vi "LDA_IP_NI-DAQmx.vi"(0 "Board type":T1=enum."NI-DAQmx", 1 "interval scanning":bool, 7 "Trigger mode":T2, 9 "output polarity":u16(ring)=1 items=["do not change", "positive", "negative"]) -> (3 "LDA Binary output":u16[][](array[numeric]), 6 "I16 TOF block (mu.s)":i16[](array[numeric])=[-338, -324, -346, -351, -326, -357, -344, -311, -375, -296], 15 "error out":errorcluster)   [LabVIEW 2012]
uses:
  Controls/Trigger_Mode.ctl
  Controls/Board_Types.ctl
  Controls/Block_start_and_end.ctl
  <vilib>/DAQmx/read.llb/DAQmx Read (Analog 2D DBL NChan NSamp).vi
  Globals/Meas_global.vi
  Globals/LDA_meas_global_1.vi
  PWA/PWAtasksGLOBAL.vi
  <vilib>/DAQmx/configure/timing.llb/DAQmx Timing (Sample Clock).vi
  <vilib>/DAQmx/create/channels.llb/DAQmx Create Channel (AI-Voltage-Basic).vi
  Globals/LDA_meas_global_2.vi
  <vilib>/DAQmx/miscellaneous.llb/DAQmx Fill In Error Info.vi
  <resource>/objmgr/daqmx.rc
panel:
  out "AI.Voltage.Rngs":dbl[](array[numeric])=[-10.0, 10.0]
  out "TotalSampPerChanAcquired":dbl=1024.0
  out "AvailSampPerChan":u32
  out "CurrReadPos":dbl=1024.0
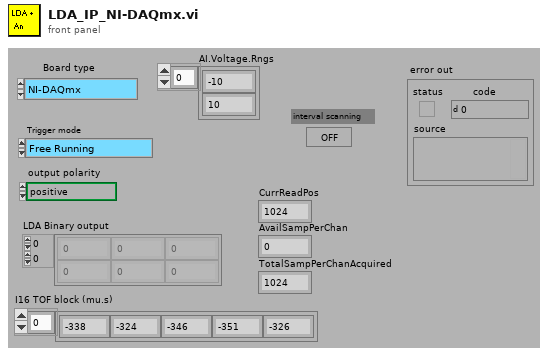
[diagram p1: front panel]
types:
  T1 = typedef "Board_Types.ctl" = enum16{"Simulate", "Local ADAM", "Server ADAM", "NI-DAQmx", "NI-DAQmxBase", "ADC488", "DT LV-link"}
  T2 = typedef "Trigger_Mode.ctl" = enum16{"Free Running", "Start on Trigger", "Trigger Every Block", "Trigger Every Sample"}
  T3 = typedef "LDA_Setup.ctl" = cluster{"dimensions":enum16{"1D", "2D"}, "Analogue Freq Multiplier":dbl}
  T4 = typedef "Ch_and_Spans.ctl" = cluster{"high limit (10V)":sgl, "low limit (-10V)":sgl, "Ch No":i16, "Var name":string, "Use Latest Calib":bool}
  T5 = typedef "Block_start_and_end.ctl" = cluster{"Started":dbl, "Ended":dbl, "Analogue Frequency Hz":dbl}
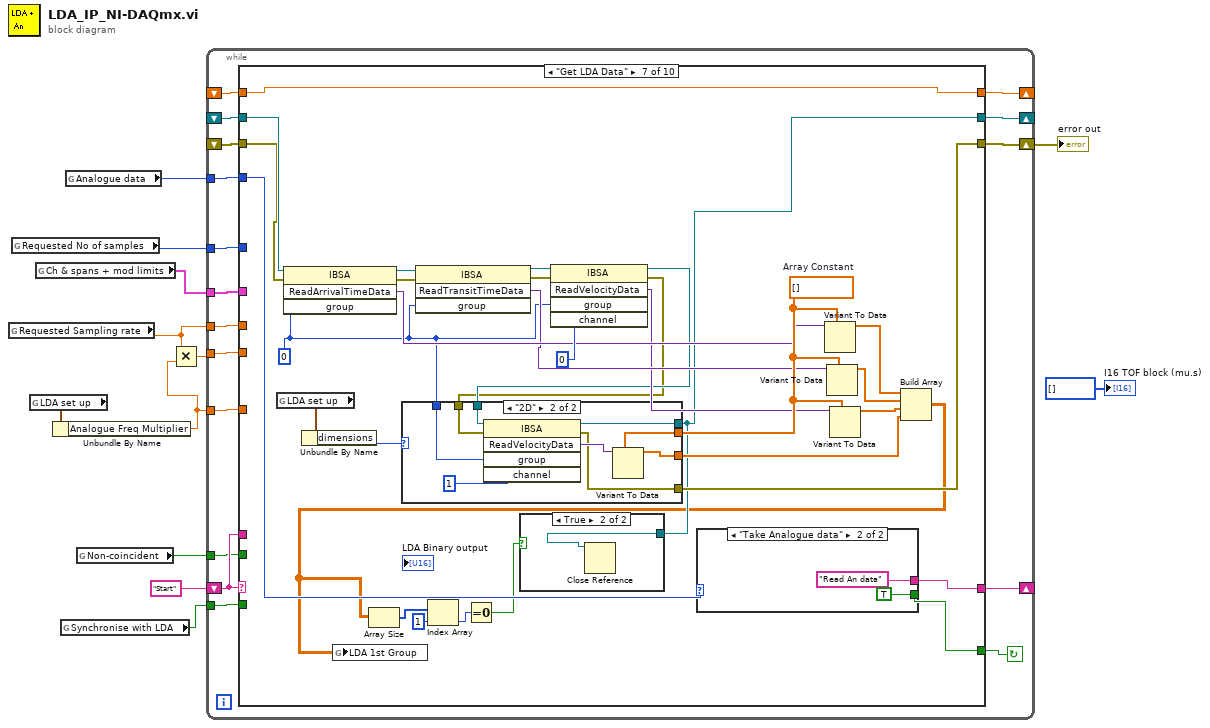
[diagram p0: block diagram]
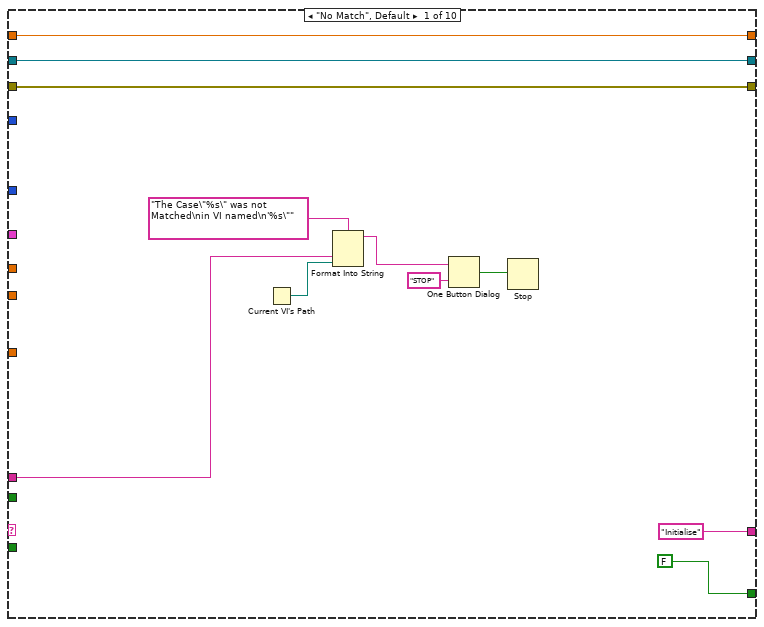
[diagram p2: hidden frame]
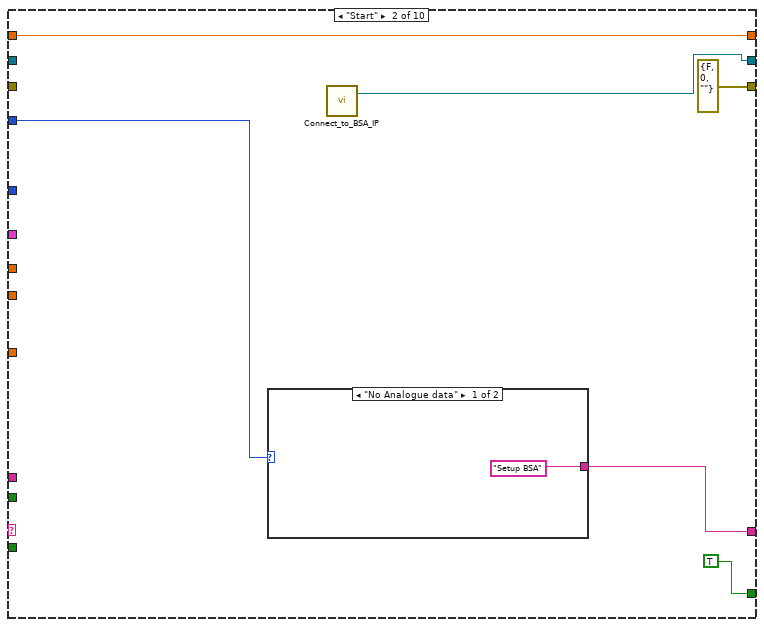
[diagram p3: hidden frame]
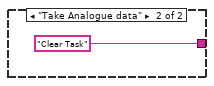
[diagram p4: hidden frame]
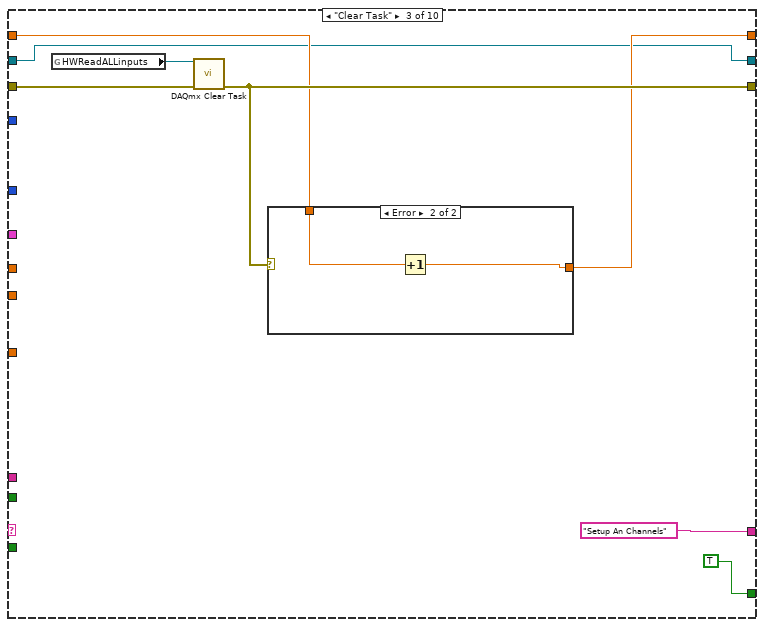
[diagram p5: hidden frame]
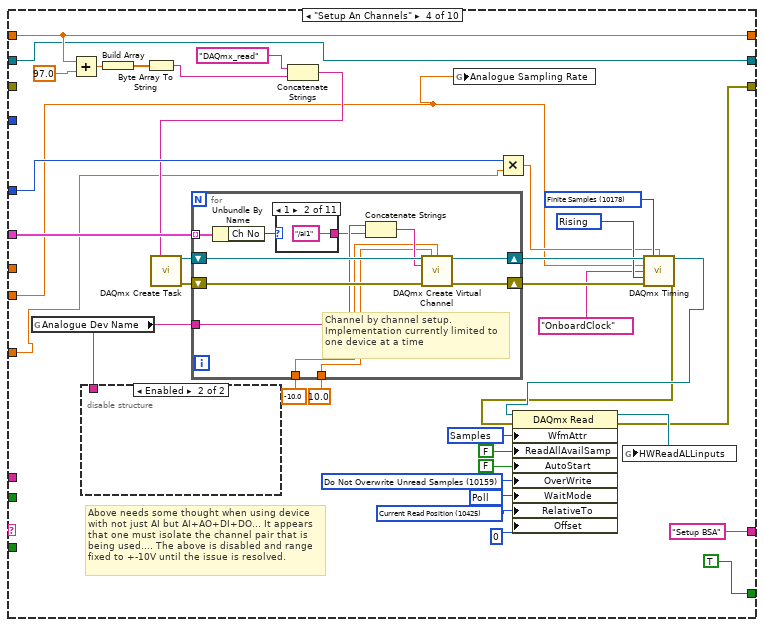
[diagram p7: hidden frame]
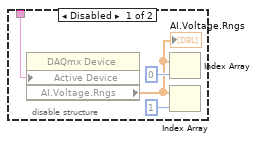
[diagram p8: hidden frame]
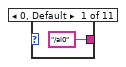
[diagram p9: hidden frame]
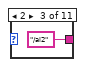
[diagram p10: hidden frame]
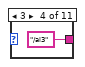
[diagram p11: hidden frame]
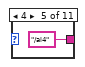
[diagram p12: hidden frame]
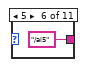
[diagram p13: hidden frame]
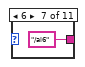
[diagram p14: hidden frame]
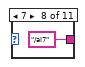
[diagram p15: hidden frame]
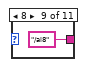
[diagram p16: hidden frame]
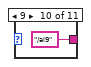
[diagram p17: hidden frame]
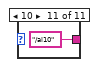
[diagram p18: hidden frame]
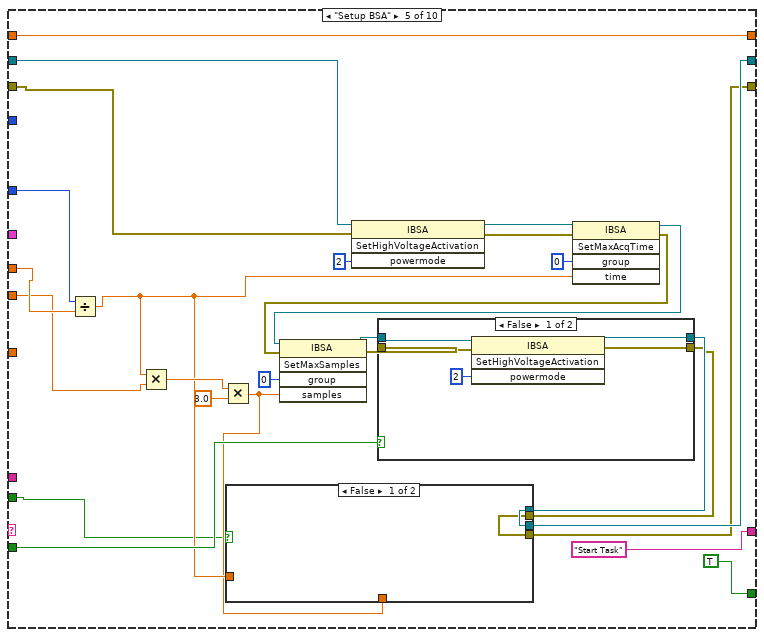
[diagram p19: hidden frame]
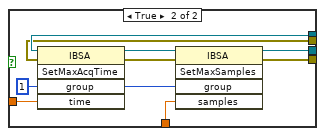
[diagram p20: hidden frame]
diagram:
  n1 = global read "Meas_global.vi" "Requested Sampling rate"() -> (w4:dbl)
  n2 = global read "Meas_global.vi" "Requested No of samples"() -> (w3:i32)
  n3 = global read "Meas_global.vi" "LDA set up"() -> (w2:T3)
  n4 = global read "Meas_global.vi" "Ch & spans + mod limits"() -> (w5:T4[])
  n5 = Unbundle By Name(w2) -> ("Analogue Freq Multiplier"=w1:dbl)
  n6 = global read "Meas_global.vi" "Synchronise with LDA"() -> (w7:bool)
  n7 = global read "Meas_global.vi" "Analogue data"() -> (w8:enum16{"No Analogue data", "Take Analogue data"})
  n8 = global read "LDA_meas_global_1.vi" "Non-coincident"() -> (w6:bool)
  n9 = Multiply(x=w4, y=w1) -> (x*y=w9:dbl)
  n10 = while {
    shift-left: "Start" -> [w27]
    shift-right: [w28] -> _
    shift-right: [w22] -> w11
    shift-left: _ -> [w26]
    tunnel: w9 -> [w25]
    tunnel: w3 -> [w24]
    tunnel: w5 -> [w23]
    shift-right: [w21] -> _
    shift-left: _ -> [w20]
    tunnel: w4 -> [w19]
    tunnel: w1 -> [w18]
    shift-right: [w16] -> _
    shift-left: _ -> [w17]
    tunnel: w8 -> [w15]
    tunnel: w7 -> [w14]
    tunnel: w6 -> [w13]
    stop <- w29 continue-if-true
    n11 = case shown="\"Get LDA Data\"" w27 {
      tunnel: [FALSE TRUE TRUE TRUE TRUE TRUE w216 w292 FALSE FALSE] -> w29
      tunnel: ["Initialise" w45 "Setup An Channels" "Setup BSA" "Start Task" w171 w236 w295 "End" "End" ("f")] -> w28
      tunnel: w27 -> [w35 _ _ _ _ _ _ _ _ _]
      tunnel: [w32 errorcluster {"status"=FALSE, "code"=0, "source"=""} ("error out") w52 w61 w125 w185 w214 w261 w311 w320] -> w22
      tunnel: w26 -> [w32 _ w53 _ w135 w173 w215 w259 w317 w320]
      tunnel: w25 -> [_ _ _ w60 w136 w181 _ _ _ _]
      tunnel: w24 -> [_ _ _ w87 w138 w183 _ _ w302 _]
      tunnel: w23 -> [_ _ _ w90 _ _ _ _ _ _]
      tunnel: [w31 w43 w51 w75 w134 w186 w235 w294 w306 w319] -> w21
      tunnel: w20 -> [w31 w43 w50 w75 w134 w186 w235 w294 w306 w319]
      tunnel: w19 -> [_ _ _ _ w137 w182 _ _ _ _]
      tunnel: w18 -> [_ _ _ w74 _ _ _ _ w305 _]
      tunnel: w17 -> [w30 _ w49 w73 w139 w179 w221 w260 w303 w318]
      tunnel: [w30 w41 w49 w73 w127 w178 w210 w258 w303 w318] -> w16
      tunnel: w15 -> [_ w46 _ _ _ w172 w217 w293 _ _]
      tunnel: w14 -> [_ _ _ _ w129 _ _ _ _ _]
      tunnel: w13 -> [_ _ _ _ w122 w170 _ _ _ _]
      frame "No Match", Default {
        n12 = Current VI's Path() -> (path=w34:path)
        n13 = Format Into String(format string="The Case\"%s\" was not Matched\nin VI named\n'%s\"" ("Format String"), w35, w34) -> (resulting string=w38:string)  [unwired: 2 in, 1 out]
        n14 = One Button Dialog(message=w38, button name ("OK")="STOP") -> (true=w36:bool)
        n15 = Stop(stop? (T)=w36) -> ()
      }
      frame "Start" {
        n16 = case shown="\"No Analogue data\"" w46 {
          tunnel: ["Setup BSA" "Clear Task"] -> w45
          frame "No Analogue data" {
          }
          frame "Take Analogue data" {
          }
        }
        n17 = call "Connect_to_BSA_IP.vi"() -> ("BSA"=w41:refnum<k7>)  [unwired: 3 out]
      }
      frame "Clear Task" {
        n18 = global read "PWAtasksGLOBAL.vi" "HWReadALLinputs"() -> (w54:refnum<k21>)
        n19 = call <vilib>:"DAQmx Clear Task.vi"("task in"=w54, "error in"=w53) -> ("error out"=w52:errorcluster)  [unwired: 13 out]
        n20 = case shown="Error" w52 {
          tunnel: [w57 w58] -> w51
          tunnel: w50 -> [w57 w59]
          frame No Error {
          }
          frame Error {
            n21 = Increment(x=w59) -> (x+1=w58:dbl)
          }
        }
      }
      frame "Setup An Channels" {
        w66 = 10425 items=["First Sample"=10424, "Current Read Position"=10425, "Reference Trigger"=10426, "First Pretrigger Sample"=10427, "Most Recent Sample"=10428] ("RelativeTo")
        w67 = 12524 items=["Wait For Interrupt"=12523, "Poll"=12524, "Yield"=12525, "Sleep"=12547] ("WaitMode")
        w68 = 10159 items=["Overwrite Unread Samples"=10252, "Do Not Overwrite Unread Samples"=10159] ("OverWrite")
        w70 = 10287 items=["Samples"=10287, "Samples and Timing"=10140, "Samples, Timing, and Attributes"=10141] ("WfmAttr")
        w89 = 10280 items=["Rising"=10280, "Falling"=10171] ("active edge")
        w93 = 10178 items=["Finite Samples"=10178, "Continuous Samples"=10123, "Hardware Timed Single Point"=12522] ("sample mode")
        # "Above needs some thought when using device with not just AI but AI+AO+DI+DO... It appears that one must isolate the channel pair that is being used.... The above is disabled and range fixed to +-10V until the issue is resolved."
        n22 = global read "PWAtasksGLOBAL.vi" "Analogue Dev Name"() -> (w82:string)
        n23 = Add(x=w75, y=97.0) -> (x+y=w80:dbl)
        n24 = disable-structure shown="Enabled" {
          disable-tunnel: w82 -> [w96 _]
          frame Disabled {
            n25 = property class="DAQmx Device"("Active Device"=w96) -> ("AI.Voltage.Rngs"=w97:dbl[])  [unwired: 2 in, 2 out]
            "AI.Voltage.Rngs" <- w97
            n26 = Index Array(array=w97, index=0) -> ()  [unwired: 1 out]
            n27 = Index Array(array=w97, index=1) -> ()  [unwired: 1 out]
          }
          frame Enabled {
          }
        }
        n28 = Build Array(w80) -> (w79:dbl[])
        n29 = Byte Array To String(unsigned byte array=w79) -> (string=w77:string)
        n30 = Concatenate Strings("DAQmx_read" ("new task name"), w77) -> (w76:string)
        n31 = call <vilib>:"DAQmx Create Task.vi"("new task name"=w76) -> ("task out"=w91:refnum<k21>, "error out"=w94:errorcluster)  [unwired: 4 in, 9 out]
        n32 = for {
          tunnel: w90 -> [w110] mode=indexing
          shift-right: [w108] -> w92
          shift-left: w91 -> [w109]
          shift-right: [w106] -> w95
          shift-left: w94 -> [w107]
          tunnel: w82 -> [w104]
          tunnel: -10.0 -> [w101]
          tunnel: 10.0 -> [w100]
          # "Channel by channel setup. Implementation currently limited to one device at a time"
          n33 = Unbundle By Name(w110) -> ("Ch No"=w105:i16)
          n34 = case shown="1" w105 {
            tunnel: ["/ai0" ("string") "/ai1" ("string") "/ai2" ("string") "/ai3" ("string") "/ai4" ("string") "/ai5" ("string") "/ai6" ("string") "/ai7" ("string") "/ai8" ("string") "/ai9" ("string") "/ai10" ("string")] -> w103
            frame 0, Default {
            }
            frame 1 {
            }
            frame 2 {
            }
            frame 3 {
            }
            frame 4 {
            }
            frame 5 {
            }
            frame 6 {
            }
            frame 7 {
            }
            frame 8 {
            }
            frame 9 {
            }
            frame 10 {
            }
          }
          n35 = Concatenate Strings(w104, w103) -> (w102:string)
          n36 = call-poly <vilib>:"DAQmx Create Virtual Channel.vi"("task in"=w109, "maximum value"=w100, "minimum value"=w101, "physical channels"=w102, "error in"=w107) -> ("task out"=w108:refnum<k21>, "error out"=w106:errorcluster)  [unwired: 4 in, 5 out]
        }
        n37 = global write "Meas_global.vi" "Analogue Sampling Rate"(w60) -> ()
        n38 = Multiply(x=w87, y=w74) -> (x*y=w86:dbl)
        n39 = call-poly <vilib>:"DAQmx Timing.vi"("task/channels in"=w92, "sample mode"=w93, "samples per channel"=w86, "rate"=w60, "source"=tag "OnboardClock", "active edge"=w89, "error in"=w95) -> ("task out"=w64:refnum<k21>, "error out"=w62:errorcluster)  [unwired: 7 out]
        n40 = property class="DAQmx Read"(reference=w64, error in=w62, "WfmAttr"=w70, "ReadAllAvailSamp"=FALSE, "AutoStart"=FALSE, "OverWrite"=w68, "WaitMode"=w67, "RelativeTo"=w66, "Offset"=0) -> (reference out=w63:refnum<k21>, error out=w61:errorcluster)
        n41 = global write "PWAtasksGLOBAL.vi" "HWReadALLinputs"(w63) -> ()
      }
      frame "Setup BSA" {
        n42 = Divide(x=w138, y=w137) -> (x/y=w124:dbl)
        n43 = Multiply(x=w124, y=w136) -> (x*y=w140:dbl)
        n44 = Multiply(x=w140, y=3.0) -> (x*y=w123:dbl)
        n45 = invoke class="IBSA" method="SetHighVoltageActivation"(reference=w139, error in=w135, "powermode"=2) -> (reference out=w146:refnum<k7>, error out=w148:errorcluster)  [unwired: 1 in, 2 out]
        n46 = invoke class="IBSA" method="SetMaxAcqTime"(reference=w146, error in=w148, "group"=0, "time"=w124) -> (reference out=w147:refnum<k7>, error out=w145:errorcluster)  [unwired: 1 in, 3 out]
        n47 = invoke class="IBSA" method="SetMaxSamples"(reference=w147, error in=w145, "group"=0, "samples"=w123) -> (reference out=w131:refnum<k7>, error out=w130:errorcluster)  [unwired: 1 in, 3 out]
        n48 = case shown="False" w129 {
          tunnel: w131 -> [w163 w168]
          tunnel: w130 -> [w162 w167]
          tunnel: [w161 w166] -> w128
          tunnel: [w160 w165] -> w126
          frame False {
            n49 = invoke class="IBSA" method="SetHighVoltageActivation"(reference=w163, error in=w162, "powermode"=2) -> (reference out=w161:refnum<k7>, error out=w160:errorcluster)  [unwired: 1 in, 2 out]
          }
          frame True {
            n50 = invoke class="IBSA" method="SetBNC"(reference=w168, error in=w167, "signal"=1) -> (reference out=w166:refnum<k7>, error out=w165:errorcluster)  [unwired: 1 in, 2 out]
          }
        }
        n51 = case shown="False" w122 {
          tunnel: w128 -> [w150 w157]
          tunnel: [w150 w155] -> w127
          tunnel: w126 -> [w149 w154]
          tunnel: [w149 w153] -> w125
          tunnel: w124 -> [_ w152]
          tunnel: w123 -> [_ w151]
          frame False {
          }
          frame True {
            w158 = 1 ("group")
            n52 = invoke class="IBSA" method="SetMaxAcqTime"(reference=w157, error in=w154, "group"=w158, "time"=w152) -> (reference out=w156:refnum<k7>, error out=w159:errorcluster)  [unwired: 1 in, 3 out]
            n53 = invoke class="IBSA" method="SetMaxSamples"(reference=w156, error in=w159, "group"=w158, "samples"=w151) -> (reference out=w155:refnum<k7>, error out=w153:errorcluster)  [unwired: 1 in, 3 out]
          }
        }
      }
      frame "Start Task" {
        n54 = Divide(x=w183, y=w182) -> (x/y=w180:dbl)
        n55 = global read "PWAtasksGLOBAL.vi" "HWReadALLinputs"() -> (w174:refnum<k21>)
        n56 = Multiply(x=w180, y=w181) -> (x*y=w177:dbl)
        n57 = Multiply(x=w177, y=3.0) -> (x*y=w176:dbl)
        n58 = case shown="\"Take Analogue data\"" w172 {
          tunnel: w173 -> [w193 w200]
          tunnel: [w192 w198] -> w185
          tunnel: w174 -> [w194 w202]
          tunnel: [w194 w201] -> w184
          tunnel: w180 -> [_ _]
          tunnel: w176 -> [_ _]
          tunnel: w179 -> [w190 w199]
          tunnel: [w191 w197] -> w178
          frame "No Analogue data" {
            n59 = invoke class="IBSA" method="StartAcq"(reference=w190, error in=w193, "waitAcqDone"=1) -> (reference out=w191:refnum<k7>, error out=w192:errorcluster)  [unwired: 1 in, 2 out]
          }
          frame "Take Analogue data" {
            n60 = stacked-sequence {
              tunnel: w202 -> [_ w205]
              tunnel: [_ w204] -> w201
              frame #0 {
                n61 = Wait (ms)(milliseconds to wait=u32 600) -> ()  [unwired: 1 out]
              }
              frame #1 {
                n62 = call <vilib>:"DAQmx Start Task.vi"("task/channels in"=w205) -> ("task out"=w204:refnum<k21>)  [unwired: 1 in, 13 out]
              }
            }
            n63 = invoke class="IBSA" method="StartAcq"(reference=w199, error in=w200, "waitAcqDone"=1) -> (reference out=w197:refnum<k7>, error out=w198:errorcluster)  [unwired: 1 in, 2 out]
          }
        }
        n64 = case shown="True" w170 {
          tunnel: ["Get LDA Data" "Get LDA data Non-coincident"] -> w171
          frame False {
          }
          frame True {
          }
        }
        n65 = global write "PWAtasksGLOBAL.vi" "HWReadALLinputs"(w184) -> ()
      }
      frame "Get LDA Data" {
        w229 = dbl[] []  # Array Constant
        w218 = 0 ("group")
        n66 = global read "Meas_global.vi" "LDA set up"() -> (w206:T3)
        n67 = invoke class="IBSA" method="ReadArrivalTimeData"(reference=w221, error in=w215, "group"=w218) -> (reference out=w234:refnum<k7>, error out=w233:errorcluster, "ReadArrivalTimeData"=w228:variant)  [unwired: 1 in, 1 out]
        n68 = Unbundle By Name(w206) -> ("dimensions"=w207:enum16{"1D", "2D"})
        n69 = invoke class="IBSA" method="ReadTransitTimeData"(reference=w234, error in=w233, "group"=w218) -> (reference out=w232:refnum<k7>, error out=w231:errorcluster, "ReadTransitTimeData"=w227:variant)  [unwired: 1 in, 1 out]
        n70 = invoke class="IBSA" method="ReadVelocityData"(reference=w232, error in=w231, "group"=w218, "channel"=0) -> (reference out=w220:refnum<k7>, error out=w219:errorcluster, "ReadVelocityData"=w226:variant)  [unwired: 1 in, 2 out]
        n71 = case shown="\"2D\"" w207 {
          tunnel: w229 -> [w243 w252]
          tunnel: [w243 w250] -> w222
          tunnel: [w244 w249] -> w210
          tunnel: w220 -> [w244 w248]
          tunnel: w219 -> [w242 w247]
          tunnel: w218 -> [_ w246]
          tunnel: [w242 w245] -> w214
          frame "1D" {
          }
          frame "2D" {
            n72 = invoke class="IBSA" method="ReadVelocityData"(reference=w248, error in=w247, "group"=w246, "channel"=1) -> (reference out=w249:refnum<k7>, error out=w245:errorcluster, "ReadVelocityData"=w251:variant)  [unwired: 1 in, 2 out]
            n73 = Variant To Data(type=w252, Variant=w251) -> (data=w250:dbl[])  [unwired: 1 in, 1 out]
          }
        }
        n74 = case shown="\"Take Analogue data\"" w217 {
          tunnel: ["End" "Read An data"] -> w236
          tunnel: [FALSE TRUE] -> w216
          frame "No Analogue data" {
          }
          frame "Take Analogue data" {
          }
        }
        n75 = Variant To Data(type=w229, Variant=w228) -> (data=w225:dbl[])  [unwired: 1 in, 1 out]
        n76 = Variant To Data(type=w229, Variant=w227) -> (data=w224:dbl[])  [unwired: 1 in, 1 out]
        n77 = Variant To Data(type=w229, Variant=w226) -> (data=w223:dbl[])  [unwired: 1 in, 1 out]
        n78 = Build Array(w225, w224, w223, w222) -> (w208:dbl[][])
        n79 = global write "LDA_meas_global_2.vi" "LDA 1st Group"(w208) -> ()
        n80 = Array Size(array=w208) -> (size(s)=w213:i32[])
        n81 = Index Array(array=w213, index=1) -> (element=w211:i32)
        n82 = Equal To 0?(x=w211) -> (x = 0?=w209:bool)
        n83 = case shown="True" w209 {
          tunnel: w210 -> [_ w237]
          frame False {
          }
          frame True {
            n84 = Close Reference(reference=w237) -> ()  [unwired: 1 in, 1 out]
          }
        }
      }
      frame "Get LDA data Non-coincident" {
        w268 = dbl[] []  # Array Constant
        w275 = 1 ("group")
        w282 = dbl[] []  # Array Constant
        w276 = 0 ("group")
        n85 = invoke class="IBSA" method="ReadArrivalTimeData"(reference=w260, error in=w259, "group"=w276) -> (reference out=w287:refnum<k7>, error out=w286:errorcluster, "ReadArrivalTimeData"=w281:variant)  [unwired: 1 in, 1 out]
        n86 = invoke class="IBSA" method="ReadTransitTimeData"(reference=w287, error in=w286, "group"=w276) -> (reference out=w285:refnum<k7>, error out=w284:errorcluster, "ReadTransitTimeData"=w280:variant)  [unwired: 1 in, 1 out]
        n87 = invoke class="IBSA" method="ReadVelocityData"(reference=w285, error in=w284, "group"=w276, "channel"=0) -> (reference out=w262:refnum<k7>, error out=w263:errorcluster, "ReadVelocityData"=w279:variant)  [unwired: 1 in, 2 out]
        n88 = invoke class="IBSA" method="ReadArrivalTimeData"(reference=w262, error in=w263, "group"=w275) -> (reference out=w270:refnum<k7>, error out=w271:errorcluster, "ReadArrivalTimeData"=w264:variant)  [unwired: 1 in, 1 out]
        n89 = invoke class="IBSA" method="ReadTransitTimeData"(reference=w270, error in=w271, "group"=w275) -> (reference out=w272:refnum<k7>, error out=w273:errorcluster, "ReadTransitTimeData"=w265:variant)  [unwired: 1 in, 1 out]
        n90 = invoke class="IBSA" method="ReadVelocityData"(reference=w272, error in=w273, "group"=w275, "channel"=1) -> (reference out=w258:refnum<k7>, error out=w261:errorcluster, "ReadVelocityData"=w266:variant)  [unwired: 1 in, 2 out]
        n91 = case shown="\"Take Analogue data\"" w293 {
          tunnel: ["End" "Read An data"] -> w295
          tunnel: [FALSE TRUE] -> w292
          frame "No Analogue data" {
          }
          frame "Take Analogue data" {
          }
        }
        n92 = Variant To Data(type=w268, Variant=w264) -> (data=w269:dbl[])  [unwired: 1 in, 1 out]
        n93 = Variant To Data(type=w268, Variant=w265) -> (data=w267:dbl[])  [unwired: 1 in, 1 out]
        n94 = Variant To Data(type=w268, Variant=w266) -> (data=w255:dbl[])  [unwired: 1 in, 1 out]
        n95 = Variant To Data(type=w282, Variant=w281) -> (data=w278:dbl[])  [unwired: 1 in, 1 out]
        n96 = Variant To Data(type=w282, Variant=w280) -> (data=w277:dbl[])  [unwired: 1 in, 1 out]
        n97 = Variant To Data(type=w282, Variant=w279) -> (data=w256:dbl[])  [unwired: 1 in, 1 out]
        n98 = Build Array(w269, w267, w255) -> (w257:dbl[][])
        n99 = global write "LDA_meas_global_2.vi" "LDA 2nd Group"(w257) -> ()
        n100 = Build Array(w278, w277, w256) -> (w254:dbl[][])
        n101 = Array Size(array=w254) -> (size(s)=w291:i32[])
        n102 = global write "LDA_meas_global_2.vi" "LDA 1st Group"(w254) -> ()
        n103 = Index Array(array=w291, index=1) -> (element=w289:i32)
        n104 = Equal To 0?(x=w289) -> (x = 0?=w288:bool)
        n105 = case shown="True" w288 {
          tunnel: w258 -> [_ w296]
          frame False {
          }
          frame True {
            n106 = Close Reference(reference=w296) -> ()  [unwired: 1 in, 1 out]
          }
        }
      }
      frame "Read An data" {
        n107 = global read "PWAtasksGLOBAL.vi" "HWReadALLinputs"() -> (w309:refnum<k21>)
        n108 = Multiply(x=w302, y=w305) -> (x*y=w304:dbl)
        n109 = call-poly <vilib>:"DAQmx Read.vi"("task/channels in"=w309, "number of samples per channel"=w304, "error in"=w317) -> ("task out"=w314:refnum<k21>, "data"=w301:dbl[][], "error out"=w308:errorcluster)  [unwired: 10 out]
        n110 = property class="DAQmx Read"(reference=w314, error in=w308) -> (reference out=w313:refnum<k21>, error out=w311:errorcluster, "CurrReadPos"=→"CurrReadPos":dbl, "AvailSampPerChan"=→"AvailSampPerChan":u32, "TotalSampPerChanAcquired"=→"TotalSampPerChanAcquired":dbl)
        n111 = global write "PWAtasksGLOBAL.vi" "HWReadALLinputs"(w313) -> ()
        n112 = global write "Meas_global.vi" "Analogue volts"(w301) -> ()
      }
      frame "Extra case" {
        (unwired) T5 {"Started"=0.0, "Ended"=0.0, "Analogue Frequency Hz"=1000.0} ("Block Timings")
      }
    }
  }
  "error out" <- w11
  "I16 TOF block (mu.s)" <- i16[] [] ("I16 TOF block (mu.s)")
